vi "Get all issues from CV.vi"() -> ()   [LabVIEW 2024]
uses:
  <vilib>/addons/_JKI.lib/REST Client/classes/REST Client/REST Client.lvclass
  CV_RESTful_Library/CV_RESTful_Lib.lvlib
  CV_Shared_Library/CV_Shared_Library.lvlib
  <vilib>/addons/_JKI.lib/Serialization/JSON/JKI JSON Serialization.lvlib
panel:
  in  "Delay Time (s)":dbl
  out "progress":i32(slide) caption="403 of 2850" scale=0.0..2850.0
  out "current file":string
  in  "dest directory":path=path "D:/Comics/data/comicvine"
  out "error out":errorcluster
  in  "issue source":path=path "D:/CV_Volumes"
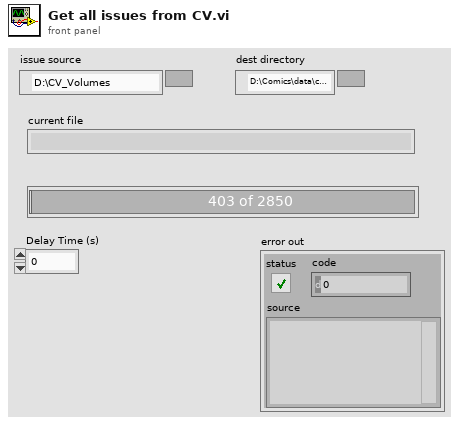
[diagram p1: front panel]
types:
  T1 = enum16{"open", "replace", "create", "open or create", "replace or create", "replace or create with confirmation"}
  T2 = typedef "local_issue.ctl" = cluster{"cover_date":timestamp, "id":i32, "cv_id":string, "name":string, "sortable_name":string, "issue_number":string, "deck":string, "description":string, "volume":T3, "store_date":timestamp, "date_last_updated":timestamp, "site_detail_url":string, "cover_url":string, "associated_images":T4[], "characters":T3[], "concepts":T3[], "creators":T5[], "storyArcs":T3[], "teams":T3[]}
  T3 = typedef "comicvine_issue.generic_credit.ctl" = cluster{"id":i32, "name":string}
  T4 = typedef "comicvine_issue.associated_image.ctl" = cluster{"original_url":string, "id":i32}
  T5 = typedef "comicvine_issue.person_credit.ctl" = cluster{"id":i32, "name":string, "role":string}
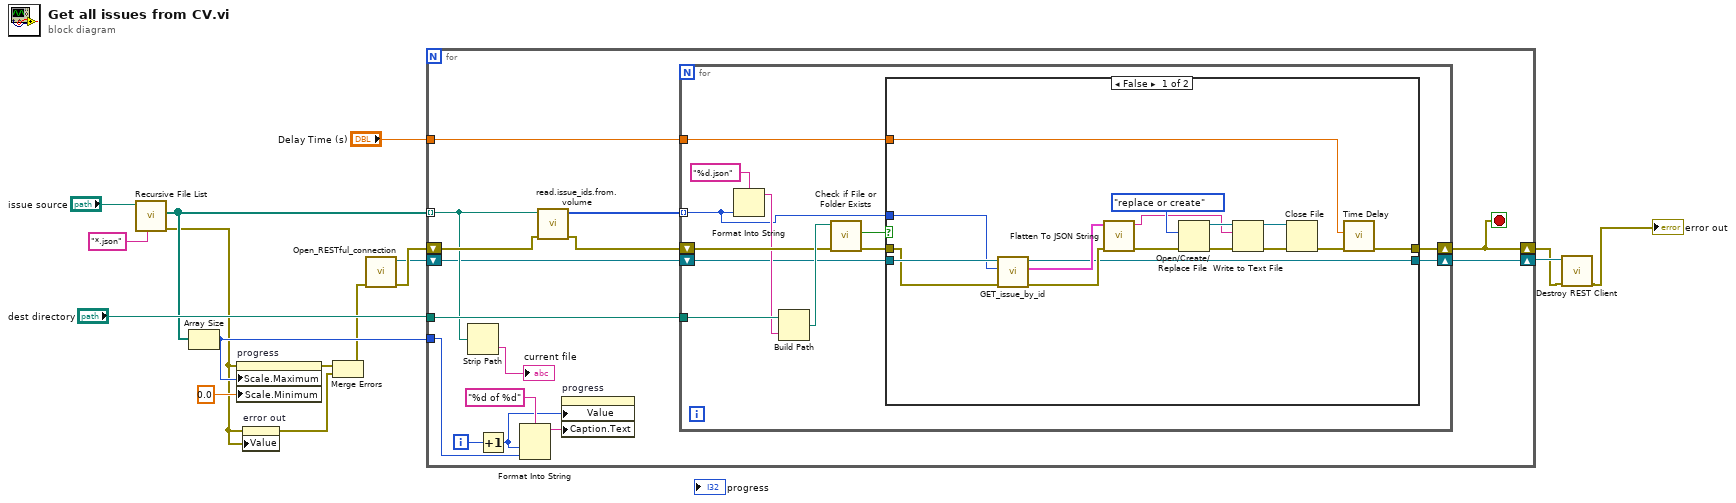
[diagram p0: block diagram]
diagram:
  n1 = call <vilib>:"Recursive File List.vi"("pattern"="*.json", "Folder Path"="issue source") -> ("error out"=w8:errorcluster, "All Files in Dir"=w10:path[])  [unwired: 5 in, 3 out]
  n2 = Array Size(array=w10) -> (size(s)=w9:i32)
  n3 = property on="progress" class="Slide (strict)"(error in=w8, "Scale.Maximum"=w9, "Scale.Minimum"=0.0 ("Scale.Range:Minimum")) -> (error out=w7:errorcluster)  [unwired: 1 in, 1 out]
  n4 = property on="error out" class="Clust (strict)"(error in=w8, "Value"=w8) -> (error out=w6:errorcluster)  [unwired: 1 in, 1 out]
  n5 = Merge Errors(w7, w6) -> (w5:errorcluster)
  n6 = call "Open_RESTful_connection.vi"("error in (no error)"=w5) -> ("error out"=w14:errorcluster, "REST Client out"=w12:refnum<class "REST Client.lvclass">)  [unwired: 9 in]
  n7 = for {
    tunnel: w10 -> [w22] mode=indexing
    shift-right: [w17] -> w2
    shift-left: w14 -> [w24]
    tunnel: "dest directory" -> [w31]
    shift-right: [w19] -> w3
    shift-left: w12 -> [w20]
    tunnel: w9 -> [w28]
    tunnel: "Delay Time (s)" -> [w18]
    i -> [w27]
    stop <- w17 stop-if-true
    n8 = Strip Path(path=w22) -> (name=→"current file":string)  [unwired: 1 out]
    n9 = Increment(x=w27) -> (x+1=w25:i32)
    n10 = Format Into String(format string="%d of %d", w25, w28) -> (resulting string=w26:string)  [unwired: 2 in, 1 out]
    n11 = call "read.issue_ids.from.volume.vi"("error in"=w24, "file (use dialog)"=w22) -> ("error out"=w23:errorcluster, "issue_ids"=w21:i32[])  [unwired: 8 in]
    n12 = property on="progress" class="Slide (strict)"("Value"=w25, "Caption.Text"=w26) -> ()  [unwired: 2 in, 2 out]
    n13 = for {
      tunnel: w31 -> [w43]
      tunnel: w21 -> [w35] mode=indexing
      shift-right: [w32] -> w19
      shift-left: w20 -> [w37]
      shift-right: [w34] -> w17
      shift-left: w23 -> [w41]
      tunnel: w18 -> [w33]
      n14 = Format Into String(format string="%d.json", w35) -> (resulting string=w39:string)  [unwired: 2 in, 1 out]
      n15 = Build Path(base path=w43, name or relative path=w39) -> (appended path=w42:path)
      n16 = call <vilib>:"Check if File or Folder Exists.vi"("error in (no error)"=w41, "path"=w42) -> ("error out"=w36:errorcluster, "file or folder exists?"=w38:bool)  [unwired: 7 in, 1 out]
      n17 = case shown="False" w38 {
        tunnel: w37 -> [w59 w61]
        tunnel: [w49 w60] -> w34
        tunnel: w36 -> [w58 w60]
        tunnel: w35 -> [w44 _]
        tunnel: w33 -> [w46 _]
        tunnel: [w45 w61] -> w32
        frame False {
          n18 = call "GET_issue_by_id.vi"("error in (no error)"=w58, "issue id"=w44, "REST Client in"=w59) -> ("error out"=w48:errorcluster, "local_issue"=w47:T2, "REST Client out"=w45:refnum<class "REST Client.lvclass">)  [unwired: 6 in]
          n19 = call <vilib>:"Flatten To JSON String.vi"("error in"=w48, "Variant"=w47) -> ("error out"=w56:errorcluster, "JSON String"=w53:string)  [unwired: 8 in]
          n20 = Open/Create/Replace File(error in=w56, operation (0:open)=T1."replace or create") -> (refnum out=w54:refnum<file>, error out=w55:errorcluster)  [unwired: 4 in, 1 out]
          n21 = Write to Text File(file (use dialog)=w54, text=w53, error in=w55) -> (refnum out=w51:refnum<file>, error out=w52:errorcluster)  [unwired: 1 in, 1 out]
          n22 = Close File(refnum=w51, error in=w52) -> (error out=w50:errorcluster)  [unwired: 1 out]
          n23 = call "Time Delay"("error in (no error)"=w50, "Delay Time (s)"=w46) -> ("error out"=w49:errorcluster)  [unwired: 9 in]
        }
        frame True {
        }
      }
    }
  }
  n24 = call-dynamic "Destroy REST Client.vi"("error in (no error)"=w2, "REST Client in"=w3) -> ("error out"=→"error out":errorcluster)  [unwired: 9 in]
